vi "Set Data Manipulation Array.vi"(8 "error in (no error)":errorcluster, 10 "Data Manipulations":refnum<class "Abstract Data Manipulator.lvclass">[](array[class]), 11 "Reference in":T1) -> (0 "error out":errorcluster, 3 "Reference out":T1)   [LabVIEW 2016, in "Impulse Data.lvclass"]
uses:
  Impulse Data.lvclass
  Instance handle.ctl
  Abstract Data Manipulator/Abstract Data Manipulator.lvclass
  Impulse Data.lvclass/Impulse Data.ctl
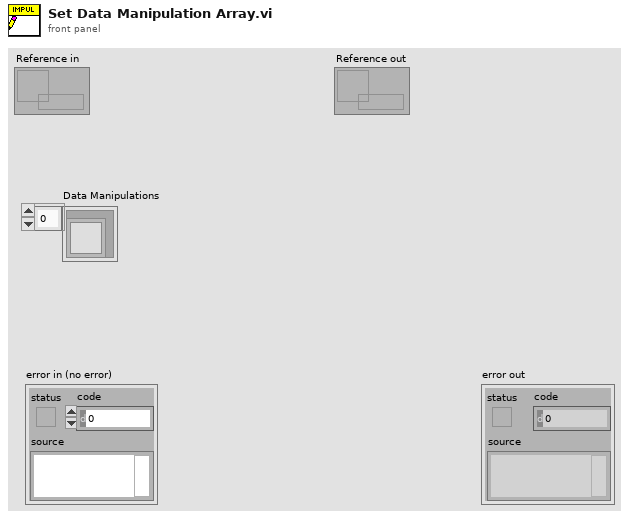
[diagram p1: front panel]
types:
  T1 = typedef "Impulse Data.lvclass/Instance handle.ctl" = refnum<data-value>
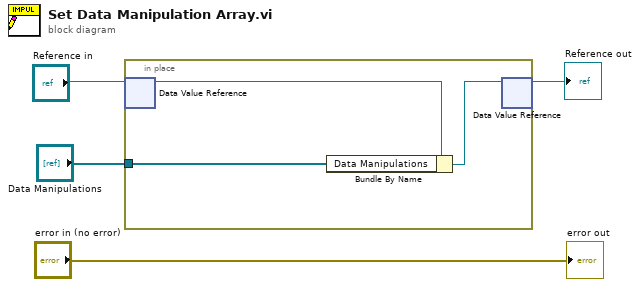
[diagram p0: block diagram]
diagram:
  n1 = in-place {
    in-place-border: "Data Manipulations" -> [w5]
    n2 = in-place-dvr #1("Reference in") -> (w7:refnum<class "Impulse Data.lvclass">)  [unwired: 1 out]
    n3 = Bundle By Name(cluster=w7, "Data Manipulations"=w5) -> (w6:refnum<class "Impulse Data.lvclass">)
    n4 = in-place-dvr #1(w6) -> (→"Reference out":T1)  [unwired: 1 out]
  }
  "error out" <- "error in (no error)"
